vi "GetCenterPoint.vi"(8 "error in (no error)":errorcluster, 11 "Control Window in":refnum<class "Control Window.lvclass">) -> (0 "error out":errorcluster, 2 "Center Point":cluster{dbl, dbl}, 3 "Control Window out":refnum<class "Control Window.lvclass">)   [LabVIEW 2015, in "Control Window.lvclass"]
uses:
  Control Window.lvclass
  Control Window.lvclass/Control Window.ctl
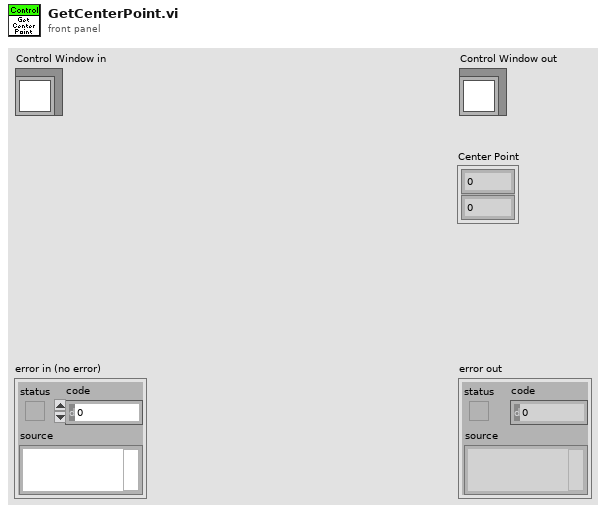
[diagram p1: front panel]
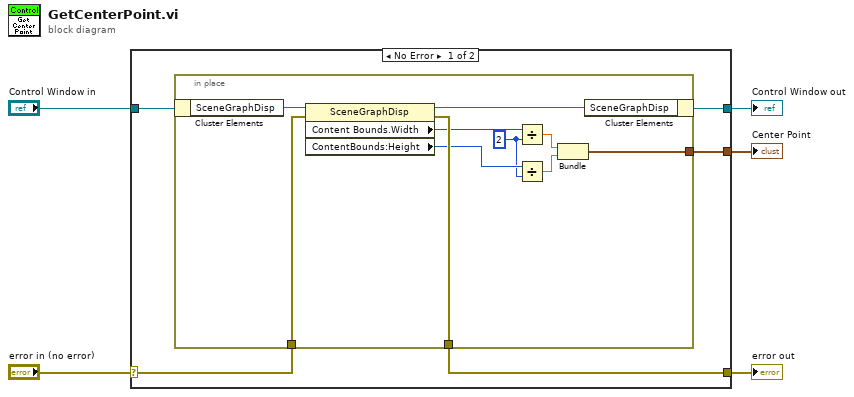
[diagram p0: block diagram]
diagram:
  n1 = case shown="No Error" "error in (no error)" {
    selector: "error in (no error)" -> [w8 w22]
    tunnel: [w7 w22] -> w4
    tunnel: [w9 w21] -> w2
    tunnel: "Control Window in" -> [w10 w21]
    tunnel: [w6 _] -> w1
    frame No Error {
      n2 = in-place {
        in-place-border: w8 -> [w18]
        in-place-border: [w17] -> w7
        in-place-border: [w11] -> w6
        w14 = u32 2 ("y")
        n3 = in-place-cluster #1(w10) -> ("SceneGraphDisp"=w20:refnum<vi>)
        n4 = property class="SceneGraphDisp"(reference=w20, error in=w18) -> (reference out=w19:refnum<vi>, error out=w17:errorcluster, "Content Bounds.Width"=w16:u32, "ContentBounds:Height"=w15:u32)
        n5 = Divide(x=w16, y=w14) -> (x/y=w13:dbl)
        n6 = Divide(x=w15, y=w14) -> (x/y=w12:dbl)
        n7 = Bundle(w13, w12) -> (w11:cluster{dbl, dbl})  [unwired: 1 in]
        n8 = in-place-cluster #1("SceneGraphDisp"=w19) -> (w9:refnum<class "Control Window.lvclass">)
      }
    }
    frame Error {
    }
  }
  "error out" <- w4
  "Control Window out" <- w2
  "Center Point" <- w1
